vi "Build Less Equal Compare Types.vi"   [LabVIEW 2021]
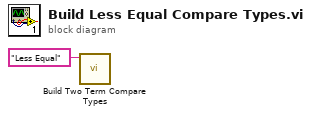
[diagram p0: block diagram]
diagram:
  n1 = call "Build Two Term Compare Types.vi"("Comparison Name"="Less Equal") -> ()  [unwired: 11 in]
